vi "Node 1 - Error Handler.vi"(8 "Error In":errorcluster, 11 "State In":T1=enum."Idle") -> (0 "Error Out":errorcluster, 3 "State Out":T1=enum."Idle")   [LabVIEW 2018]
uses:
  Node 1 - States.ctl
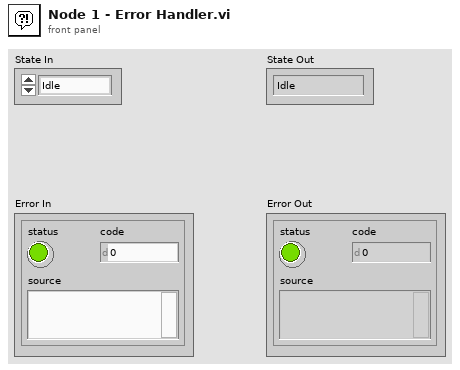
[diagram p1: front panel]
types:
  T1 = typedef "Node 1 - States.ctl" = enum16{"Initialize", "Read Sensors", "Toggle Pump", "Read HB", "Safe State", "Evaluate Error", "Log Error", "Reset Wifi", "Idle"}
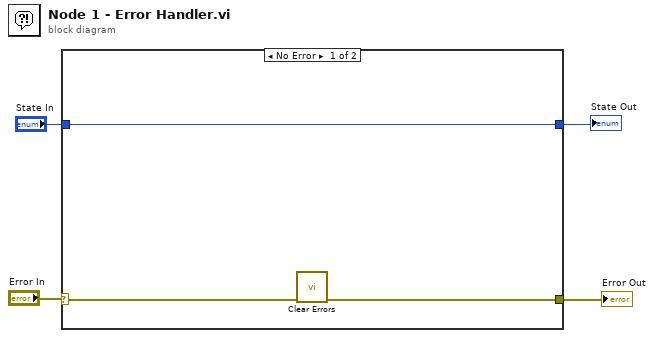
[diagram p0: block diagram]
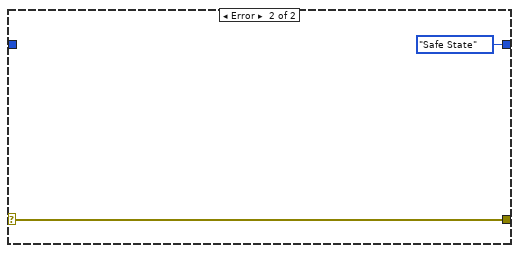
[diagram p2: hidden frame]
diagram:
  n1 = case shown="No Error" "Error In" {
    selector: "Error In" -> [w7 w9]
    tunnel: [w5 w9] -> w3
    tunnel: "State In" -> [w6 _]
    tunnel: [w6 Node_1_-_States."Safe State" ("State In")] -> w1
    frame No Error {
      n2 = call <vilib>:"Clear Errors.vi"("error in (no error)"=w7) -> ("error out"=w5:errorcluster)  [unwired: 5 in, 1 out]
    }
    frame Error {
    }
  }
  "State Out" <- w1
  "Error Out" <- w3
